vi "Main Generador N03.vi"(8 "error in":errorcluster, 11 "Network Path":string="192.168.169.1") -> (0 "error out":errorcluster, 2 "Equipo conectado":bool)   [LabVIEW 2015]
uses:
  Controles/Hora y Fecha.ctl
panel:
  in  "Stop Button":bool
  out "Alarmas":string
  out "Time Stamp":T1 format="%<%H:%M                            %x>T\n"
  out "I3_IEE_THD%":sgl format="%.3f"
  out "I2_IEE_THD%":sgl format="%.3f"
  out "I1_IEE_THD%":sgl format="%.3f"
  out "V3_V1_IEE_THD%":sgl format="%.3f"
  out "V2_V3_IEE_THD%":sgl format="%.3f"
  out "V1_V2_IEE_THD%":sgl format="%.3f"
  out "I3_Crest_Factor":sgl format="%.3f"
  out "I2_Crest_Factor":sgl format="%.3f"
  out "I1_Crest_Factor":sgl format="%.3f"
  out "V3_V1_Crest_Factor":sgl format="%.3f"
  out "V2_V3_Crest_Factor":sgl format="%.3f"
  out "V1_V2_Crest_Factor":sgl format="%.3f"
  out "Total_Disp_PF":sgl format="%.3f"
  out "Total_True_PF":sgl format="%.3f"
  out "Total_kVA":sgl format="%.3f"
  out "Total_kVAR":sgl format="%.3f"
  out "Total_kW":sgl format="%.3f"
  out "Frequency_Hz":sgl format="%.3f"
  out "I3_Amps":sgl format="%.3f"
  out "I2_Amps":sgl format="%.3f"
  out "I1_Amps":sgl format="%.3f"
  out "V3_V1_Volts":sgl format="%.3f"
  out "V2_V3_Volts":sgl format="%.3f"
  out "V1_V2_Volts":sgl format="%.3f"
  # "G03"
  # "Generador Diesel N°3 Popa"
  # "Hora:"
  # "Fecha:"
  # "GENERAL"
  # "CALIDAD DE ENERGIA"
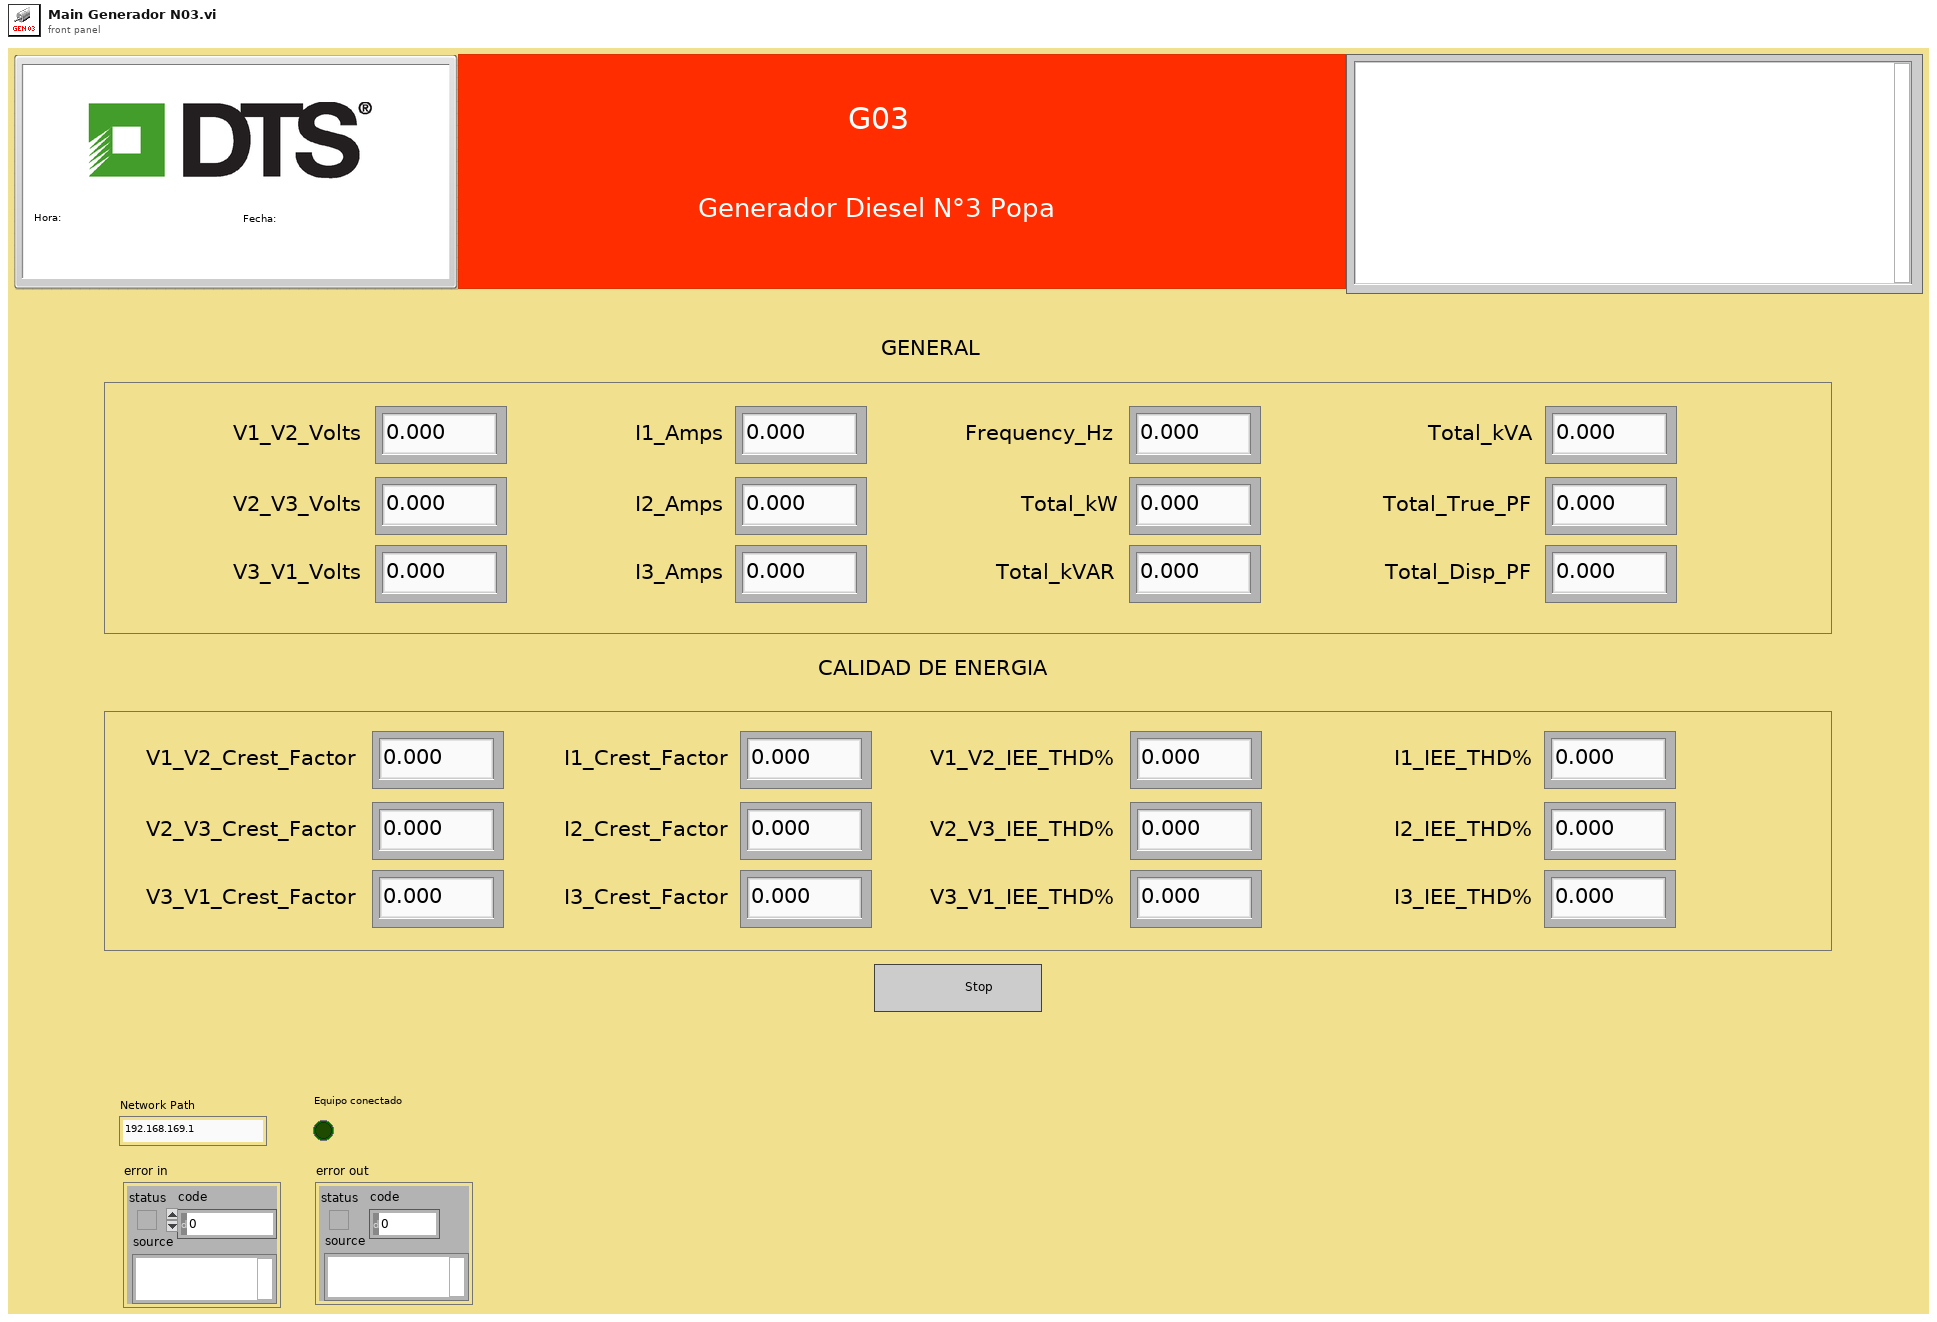
[diagram p1: front panel]
types:
  T1 = typedef "Hora y Fecha.ctl" = timestamp
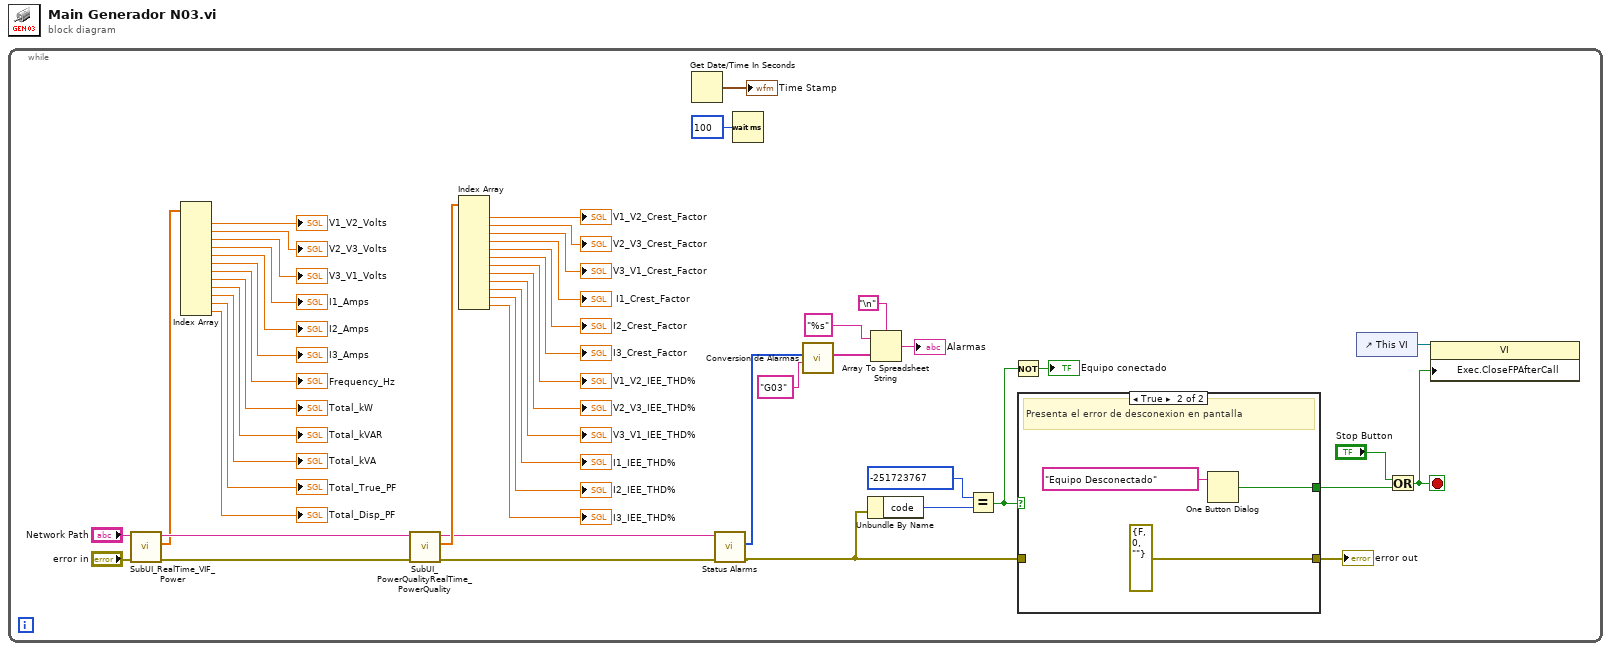
[diagram p0: block diagram]
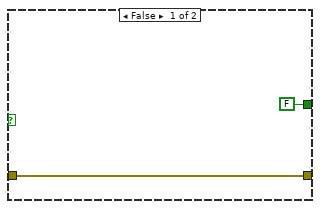
[diagram p2: hidden frame]
diagram:
  n1 = while {
    stop <- w1 stop-if-true
    n2 = call "SubUI_RealTime_VIF_Power.vi"("error in"="error in", "Network Path"="Network Path") -> ("error out"=w50:errorcluster, "Data array"=w44:sgl[], "Network Path out"=w45:string)  [unwired: 7 in]
    n3 = Index Array(array=w44) -> (element #1=→"V1_V2_Volts":sgl, element #2=→"V2_V3_Volts":sgl, element #3=→"V3_V1_Volts":sgl, element #4=→"I1_Amps":sgl, element #5=→"I2_Amps":sgl, element #6=→"I3_Amps":sgl, element #7=→"Frequency_Hz":sgl, element #8=→"Total_kW":sgl, element #9=→"Total_kVAR":sgl, element #10=→"Total_kVA":sgl, element #11=→"Total_True_PF":sgl, element #12=→"Total_Disp_PF":sgl)  [unwired: 12 in]
    n4 = call "SubUI_PowerQualityRealTime_PowerQuality.vi"("error in"=w50, "Network Path In"=w45) -> ("error out"=w12:errorcluster, "Data Array"=w31:sgl[], "Network Path Out"=w13:string)  [unwired: 7 in]
    n5 = Index Array(array=w31) -> (element #1=→"V1_V2_Crest_Factor":sgl, element #2=→"V2_V3_Crest_Factor":sgl, element #3=→"V3_V1_Crest_Factor":sgl, element #4=→"I1_Crest_Factor":sgl, element #5=→"I2_Crest_Factor":sgl, element #6=→"I3_Crest_Factor":sgl, element #7=→"V1_V2_IEE_THD%":sgl, element #8=→"V2_V3_IEE_THD%":sgl, element #9=→"V3_V1_IEE_THD%":sgl, element #10=→"I1_IEE_THD%":sgl, element #11=→"I2_IEE_THD%":sgl, element #12=→"I3_IEE_THD%":sgl)  [unwired: 12 in]
    n6 = Get Date/Time In Seconds() -> (seconds since 1Jan1904=→"Time Stamp":timestamp)
    n7 = call "Status Alarms.vi"("error in"=w12, "Network Path In"=w13) -> ("error out"=w11:errorcluster, "Data"=w9:i16[])  [unwired: 7 in, 1 out]
    n8 = Wait (ms)(milliseconds to wait=u32 100) -> ()  [unwired: 1 out]
    n9 = call "Conversion de Alarmas.vi"("Fuente"="G03", "Data Alarms"=w9) -> ("Description Alarms"=w8:string[])  [unwired: 9 in]
    n10 = Unbundle By Name(w11) -> ("code"=w18:i32)
    n11 = Array To Spreadsheet String(delimiter (Tab)="\n", array=w8, 3:"%s" ("format string")) -> (spreadsheet string=→"Alarmas":string)
    n12 = Equal?(x=-251723767, y=w18) -> (x = y?=w14:bool)
    n13 = Not(x=w14) -> (.not. x?=→"Equipo conectado":bool)
    n14 = case shown="True" w14 {
      tunnel: w11 -> [w52 _]
      tunnel: [w52 errorcluster {"status"=FALSE, "code"=0, "source"=""} ("error constant")] -> w16
      tunnel: [FALSE ("true") w53] -> w4
      frame False {
      }
      frame True {
        # "Presenta el error de desconexion en pantalla"
        n15 = One Button Dialog(message="Equipo Desconectado") -> (true=w53:bool)  [unwired: 1 in]
      }
    }
    "error out" <- w16
    n16 = control-ref of="This VI"() -> (w2:refnum<vi>)
    n17 = Or(x="Stop Button", y=w4) -> (x .or. y?=w1:bool)
    n18 = property class="VI"(reference=w2, "Exec.CloseFPAfterCall"=w1) -> ()  [unwired: 1 in, 2 out]
  }
